vi "Solution part 2.vi"(11 "data?":bool) -> (3 "Distance":i32)   [LabVIEW 2020]
uses:
  Direction.ctl
  WindStar.ctl
panel:
  out "Waypoint Relative Position":T1
  out "Ship Position":T1
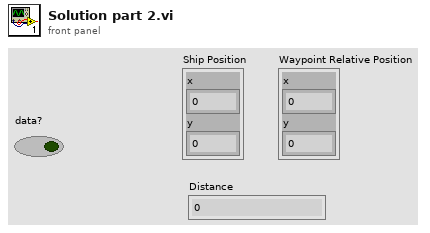
[diagram p1: front panel]
types:
  T1 = typedef "Direction.ctl" = cluster{"x":i32, "y":i32}
  T2 = typedef "WindStar.ctl" = enum16{"N", "NE", "E", "SE", "S", "SW", "W", "NW", "F", "R", "L"}
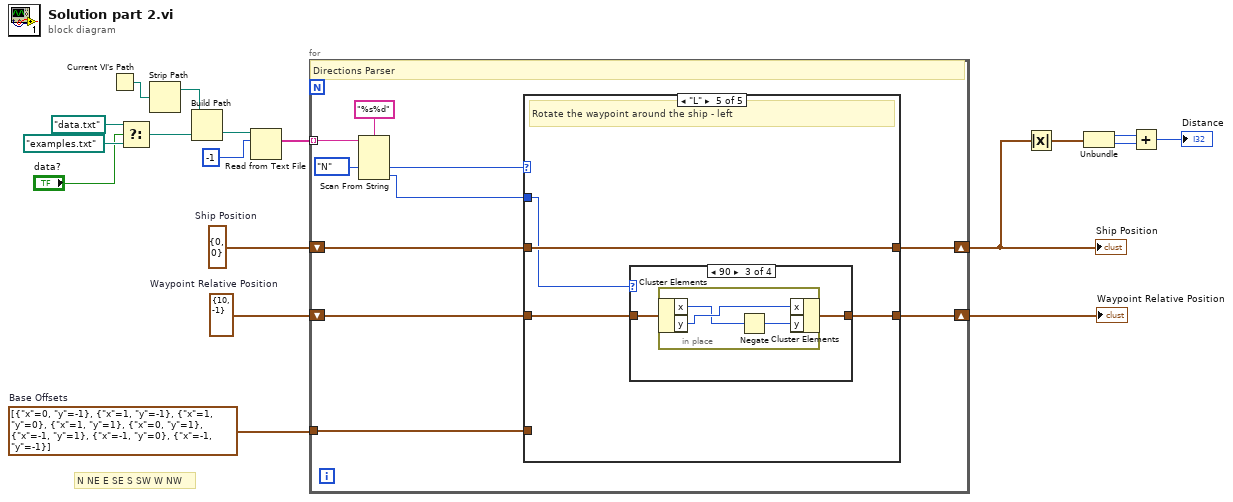
[diagram p0: block diagram]
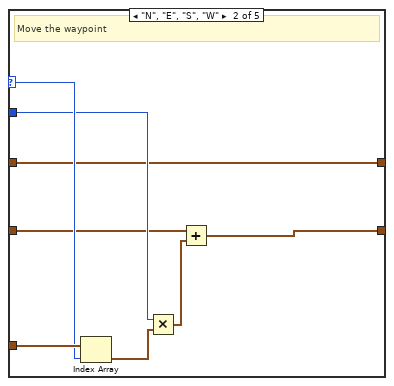
[diagram p3: hidden frame]
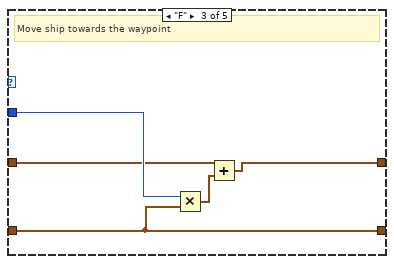
[diagram p4: hidden frame]
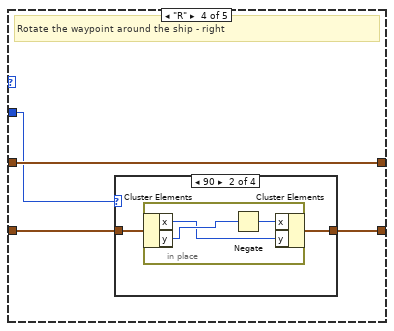
[diagram p5: hidden frame]
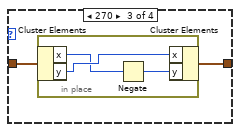
[diagram p7: hidden frame]
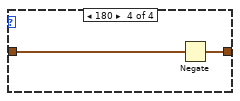
[diagram p8: hidden frame]
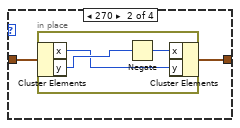
[diagram p10: hidden frame]
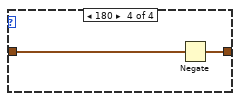
[diagram p11: hidden frame]
diagram:
  w2 = T1 {"x"=10, "y"=-1}  # Waypoint Relative Position
  w8 = T1[] [{"x"=0, "y"=-1}, {"x"=1, "y"=-1}, {"x"=1, "y"=0}, {"x"=1, "y"=1}, {"x"=0, "y"=1}, {"x"=-1, "y"=1}, {"x"=-1, "y"=0}, {"x"=-1, "y"=-1}]  # Base Offsets
  w9 = T1 {"x"=0, "y"=0}  # Ship Position
  # "N NE E SE S SW W NW"
  n1 = Current VI's Path() -> (path=w15:path)
  n2 = Select(t=path "data.txt", s="data?", f=path "examples.txt") -> (s? t:f=w16:path)
  n3 = Strip Path(path=w15) -> (stripped path=w14:path)  [unwired: 1 out]
  n4 = Build Path(base path=w14, name or relative path=w16) -> (appended path=w13:path)
  n5 = Read from Text File(file (use dialog)=w13, count=-1) -> (text=w10:string[])  [unwired: 2 in, 3 out]
  n6 = for {
    tunnel: w10 -> [w28] mode=indexing
    shift-right: [w23] -> w7
    shift-left: w9 -> [w26]
    tunnel: w8 -> [w25]
    shift-right: [w19] -> w1
    shift-left: w2 -> [w20]
    # "Directions Parser"
    n7 = Scan From String(format string="%s%d", input string=w28, default 1=WindStar."N") -> (output 1=w21:T2, output 2=w24:i32)  [unwired: 3 in, 3 out]
    n8 = case shown="\"L\"" w21 {
      selector: w21 -> [_ w37 _ _ _]
      tunnel: w26 -> [w30 w33 w42 w47 w64]
      tunnel: w25 -> [_ w38 _ _ _]
      tunnel: w24 -> [_ w35 w43 w46 w63]
      tunnel: [w30 w33 w40 w47 w64] -> w23
      tunnel: w20 -> [w29 w34 w39 w45 w62]
      tunnel: [w29 w32 w39 w44 w61] -> w19
      frame Default {
      }
      frame "N", "E", "S", "W" {
        # "Move the waypoint"
        n9 = Index Array(array=w38, index=w37) -> (element=w36:T1)
        n10 = Multiply(x=w35, y=w36) -> (x*y=w31:T1)
        n11 = Add(x=w34, y=w31) -> (x+y=w32:T1)
      }
      frame "F" {
        # "Move ship towards the waypoint"
        n12 = Multiply(x=w43, y=w39) -> (x*y=w41:T1)
        n13 = Add(x=w42, y=w41) -> (x+y=w40:T1)
      }
      frame "R" {
        # "Rotate the waypoint around the ship - right"
        n14 = case shown="90" w46 {
          tunnel: w45 -> [w48 w50 w55 w60]
          tunnel: [w48 w49 w54 w59] -> w44
          frame 0, Default {
          }
          frame 90 {
            n15 = in-place {
              n16 = in-place-cluster #1(w50) -> ("x"=w52:i32, "y"=w53:i32)
              n17 = Negate(x=w53) -> (-x=w51:i32)
              n18 = in-place-cluster #1("x"=w51, "y"=w52) -> (w49:T1)
            }
          }
          frame 270 {
            n19 = in-place {
              n20 = in-place-cluster #2(w55) -> ("x"=w57:i32, "y"=w58:i32)
              n21 = Negate(x=w57) -> (-x=w56:i32)
              n22 = in-place-cluster #2("x"=w58, "y"=w56) -> (w54:T1)
            }
          }
          frame 180 {
            n23 = Negate(x=w60) -> (-x=w59:T1)
          }
        }
      }
      frame "L" {
        # "Rotate the waypoint around the ship - left"
        n24 = case shown="90" w63 {
          tunnel: w62 -> [w65 w67 w72 w77]
          tunnel: [w65 w66 w71 w76] -> w61
          frame 0, Default {
          }
          frame 270 {
            n25 = in-place {
              n26 = in-place-cluster #3(w67) -> ("x"=w69:i32, "y"=w70:i32)
              n27 = Negate(x=w70) -> (-x=w68:i32)
              n28 = in-place-cluster #3("x"=w68, "y"=w69) -> (w66:T1)
            }
          }
          frame 90 {
            n29 = in-place {
              n30 = in-place-cluster #4(w72) -> ("x"=w74:i32, "y"=w75:i32)
              n31 = Negate(x=w74) -> (-x=w73:i32)
              n32 = in-place-cluster #4("x"=w75, "y"=w73) -> (w71:T1)
            }
          }
          frame 180 {
            n33 = Negate(x=w77) -> (-x=w76:T1)
          }
        }
      }
    }
  }
  "Ship Position" <- w7
  "Waypoint Relative Position" <- w1
  n34 = Absolute Value(x=w7) -> (abs(x)=w6:T1)
  n35 = Unbundle(w6) -> ("x"=w5:i32, "y"=w4:i32)
  n36 = Add(x=w5, y=w4) -> (x+y=→"Distance":i32)
